vi "Obtain Broadcast Events.vi"(8 "error in":errorcluster, 10 "Create New? (F)":bool) -> (0 "error out":errorcluster, 2 "Panther Dashboard Broadcast Events":T1)   [LabVIEW 2019, in "Panther Dashboard.lvlib"]
doc: "This VI Obtains/Creates the Broadcast events that will be used for other modules to register to receive messages from the module that owns this VI.\n\n<b>NOTE</b>: The contents of this VI are automatically generated and modified by the <b>Tools > Delacor > DQMH</b> utilities. Consider using those utilities instead of making your own modifications to this VI.\n_____\nBased on DQMH Project Template 6.1.0.94."
uses:
  Panther Dashboard.lvlib
  Broadcast Events--cluster.ctl
  Did Init Argument--cluster.ctl
  Status Updated Argument--cluster.ctl
  Error Reported Argument--cluster.ctl
  Stop Argument--cluster.ctl
  Get Module Execution Status Argument--cluster.ctl
  References Updated Argument--cluster.ctl
  Module type--enum.ctl
  Project References--cluster.ctl
  Progress updated Argument--cluster.ctl
  Scale Updated Argument--cluster.ctl
  Connector Pane Updated Argument--cluster.ctl
  Documentation Updated Argument--cluster.ctl
  Documentation--cluster.ctl
  Module Type Updated Argument--cluster.ctl
  Project Description Updated Argument--cluster.ctl
panel:
  # "NOTE: The contents of this VI are automatically generated and modified by the Tools > Delacor > DQMH utilities. Consider using those utilities instead of making your own modifications to this VI."
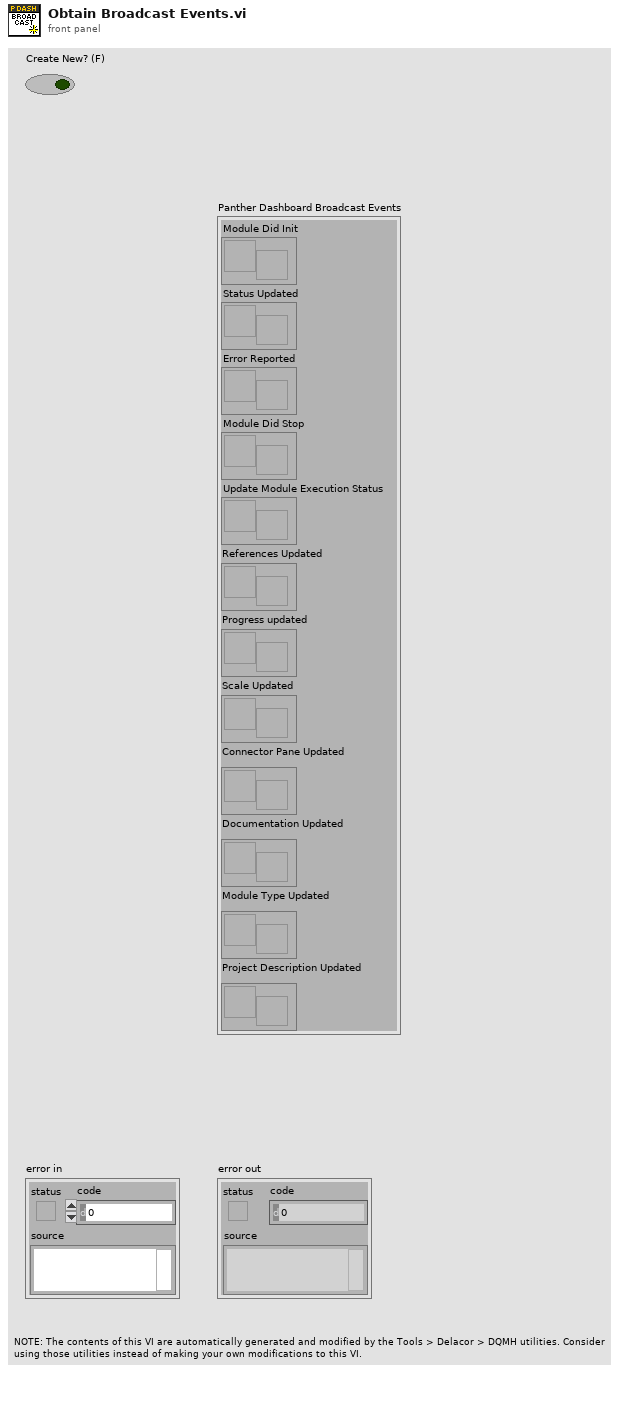
[diagram p1: front panel]
types:
  T1 = typedef "Panther Dashboard.lvlib/Broadcast Events--cluster.ctl" = cluster{"Module Did Init":refnum<user-event>, "Status Updated":refnum<user-event>, "Error Reported":refnum<user-event>, "Module Did Stop":refnum<user-event>, "Update Module Execution Status":refnum<user-event>, "References Updated":refnum<user-event>, "Progress updated":refnum<user-event>, "Scale Updated":refnum<user-event>, "Connector Pane Updated":refnum<user-event>, "Documentation Updated":refnum<user-event>, "Module Type Updated":refnum<user-event>, "Project Description Updated":refnum<user-event>}
  T2 = typedef "Panther Dashboard.lvlib/Project Description Updated Argument--cluster.ctl" = cluster{"Project Description":string}
  T3 = typedef "Panther Dashboard.lvlib/Module Type Updated Argument--cluster.ctl" = cluster{"Module Type":T4}
  T4 = typedef "Panther Dashboard.lvlib/Module type--enum.ctl" = enum16{"Singleton", "Cloneable"}
  T5 = typedef "Panther Dashboard.lvlib/Documentation Updated Argument--cluster.ctl" = cluster{"Documentation":T6}
  T6 = typedef "Panther Dashboard.lvlib/Documentation--cluster.ctl" = cluster{"Module Description":string, "Event Description":string}
  T7 = typedef "Panther Dashboard.lvlib/Connector Pane Updated Argument--cluster.ctl" = cluster{"Event Connector Pane":picture}
  T8 = typedef "Panther Dashboard.lvlib/Scale Updated Argument--cluster.ctl" = cluster{"Scale Max":i32}
  T9 = typedef "Panther Dashboard.lvlib/Progress updated Argument--cluster.ctl" = cluster{"Progress":u16}
  T10 = typedef "Panther Dashboard.lvlib/References Updated Argument--cluster.ctl" = cluster{"Modules":refnum<vi>[], "Modules Types":T4[], "Dependencies":bool[], "References":T11}
  T11 = typedef "Panther Dashboard.lvlib/Project References--cluster.ctl" = cluster{"Project Ref":refnum<vi>, "Project Name":string, "Target App Ref":refnum<vi>, "Target Ref":refnum<vi>, "Target Name":string, "Main App Ref":refnum<vi>}
  T12 = typedef "Panther Dashboard.lvlib/Get Module Execution Status Argument--cluster.ctl" = cluster{"Running?":bool}
  T13 = typedef "Panther Dashboard.lvlib/Stop Argument--cluster.ctl" = cluster{"Origin":string, "Exit via Stop Module Req?":bool, "Wait for Module to stop?":bool}
  T14 = typedef "Panther Dashboard.lvlib/Error Reported Argument--cluster.ctl" = cluster{"Error":errorcluster, "Additional Information":string, "Module Name":string}
  T15 = typedef "Panther Dashboard.lvlib/Status Updated Argument--cluster.ctl" = cluster{"Status":string}
  T16 = typedef "Panther Dashboard.lvlib/Did Init Argument--cluster.ctl" = cluster{"Init?":bool, "Info":string}
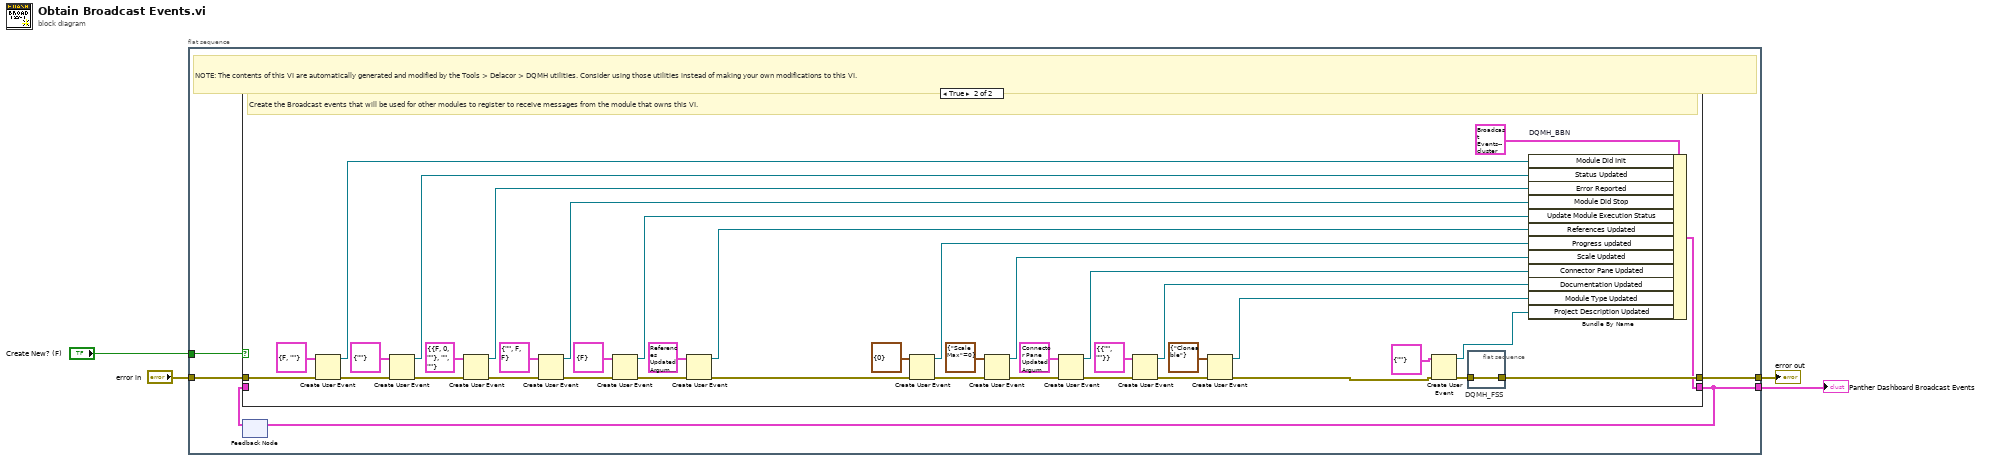
[diagram p0: block diagram]
diagram:
  n1 = flat-sequence {
    tunnel: [w9] -> w4
    tunnel: "error in" -> [w8]
    tunnel: [w6] -> w2
    tunnel: "Create New? (F)" -> [w5]
    frame #0 {
      # "NOTE: The contents of this VI are automatically generated and modified by the Tools > Delacor > DQMH utilities. Consider using those utilities instead of making your own modifications to this VI."
      n2 = feedback #1() -> (w7:T1)  [unwired: 1 in]
      n3 = case shown="True" w5 {
        tunnel: [w11 w46] -> w9
        tunnel: w8 -> [w11 w51]
        tunnel: [w10 w35] -> w6
        tunnel: w7 -> [w10 _]
        frame False {
          # "Obtain the Broadcast events that were created in a previous call to this VI."
        }
        frame True {
          # "Create the Broadcast events that will be used for other modules to register to receive messages from the module that owns this VI."
          n4 = Create User Event(user event datatype=T16 {"Init?"=FALSE, "Info"=""} ("Did Init Argument"), error in=w51) -> (user event=w36:refnum<user-event>, error out=w50:errorcluster)
          n5 = Create User Event(user event datatype=T15 {"Status"=""} ("Status Updated Argument"), error in=w50) -> (user event=w32:refnum<user-event>, error out=w49:errorcluster)
          n6 = Create User Event(user event datatype=T14 {"Error"={"status"=FALSE, "code"=0, "source"=""}, "Additional Information"="", "Module Name"=""} ("Error Reported Argument"), error in=w49) -> (user event=w30:refnum<user-event>, error out=w48:errorcluster)
          n7 = Create User Event(user event datatype=T13 {"Origin"="", "Exit via Stop Module Req?"=FALSE, "Wait for Module to stop?"=FALSE} ("Stop Argument"), error in=w48) -> (user event=w28:refnum<user-event>, error out=w47:errorcluster)
          n8 = Create User Event(user event datatype=T12 {"Running?"=FALSE} ("Get Module Execution Status Argument"), error in=w47) -> (user event=w27:refnum<user-event>, error out=w45:errorcluster)
          n9 = Create User Event(user event datatype=T10 {"Modules"=[], "Modules Types"=[], "Dependencies"=[], "References"={"Project Ref"=refnum, "Project Name"="", "Target App Ref"=refnum, "Target Ref"=refnum, "Target Name"="", "Main App Ref"=refnum}} ("References Updated Argument"), error in=w45) -> (user event=w25:refnum<user-event>, error out=w44:errorcluster)
          n10 = Create User Event(user event datatype=T9 {"Progress"=0} ("Progress updated Argument"), error in=w44) -> (user event=w23:refnum<user-event>, error out=w43:errorcluster)
          n11 = Create User Event(user event datatype=T8 {"Scale Max"=0} ("Scale Updated Argument"), error in=w43) -> (user event=w21:refnum<user-event>, error out=w42:errorcluster)
          n12 = Create User Event(user event datatype=T7 {"Event Connector Pane"=bytes[0]} ("Connector Pane Updated Argument"), error in=w42) -> (user event=w19:refnum<user-event>, error out=w41:errorcluster)
          n13 = Create User Event(user event datatype=T5 {"Documentation"={"Module Description"="", "Event Description"=""}} ("Documentation Updated Argument"), error in=w41) -> (user event=w17:refnum<user-event>, error out=w40:errorcluster)
          n14 = Create User Event(user event datatype=T3 {"Module Type"=enum."Cloneable"} ("Module Type Updated Argument"), error in=w40) -> (user event=w15:refnum<user-event>, error out=w39:errorcluster)
          n15 = Create User Event(user event datatype=T2 {"Project Description"=""} ("Project Description Updated Argument"), error in=w39) -> (user event=w13:refnum<user-event>, error out=w38:errorcluster)
          n16 = flat-sequence "DQMH_FSS" {
            tunnel: w38 -> [w52]
            tunnel: [w52] -> w46
            frame #0 {
            }
          }
          n17 = Bundle By Name "DQMH_BBN"(cluster=T1 {"Module Did Init"=refnum, "Status Updated"=refnum, "Error Reported"=refnum, "Module Did Stop"=refnum, "Update Module Execution Status"=refnum, "References Updated"=refnum, "Progress updated"=refnum, "Scale Updated"=refnum, "Connector Pane Updated"=refnum, "Documentation Updated"=refnum, "Module Type Updated"=refnum, "Project Description Updated"=refnum} ("output cluster"), "Module Did Init"=w36, "Status Updated"=w32, "Error Reported"=w30, "Module Did Stop"=w28, "Update Module Execution Status"=w27, "References Updated"=w25, "Progress updated"=w23, "Scale Updated"=w21, "Connector Pane Updated"=w19, "Documentation Updated"=w17, "Module Type Updated"=w15, "Project Description Updated"=w13) -> (w35:T1)
        }
      }
      n18 = feedback-in #1(w6) -> ()
    }
  }
  "Panther Dashboard Broadcast Events" <- w2
  "error out" <- w4
